vi "read from wavemeter_clock_2015.vi"(2 "error in (no error)":errorcluster, 3 "Single Measurement?":bool, 4 "Select Port":refnum<visa-resource-name>="COM4") -> (0 "error out":errorcluster, 1 "frequency":string="010849.313", 5 "Units":string=" cm-1")   [LabVIEW 2016]
uses:
  <vilib>/Instr/_visa.llb/VISA Configure Serial Port (Instr).vi
panel:
  in  "Case Constant\n(See Context Help) 2":bool=TRUE
  in  "Case Constant\n(See Context Help)":bool
  in  "termination char\n(0xA = '\\n' = LF)":u8=10 format="%.0x"
  in  "Tab Control":enum32{"Wavelength Monitor", "Nuts and Bolts"}(tab)
  out "Timestamp":string="17:39:12"
  out "Frequency":string="325253.97  GHz"
  out "Wavenumber":string="921.7173  nm"
  out "Wavelength":string="+010849.313  cm-1"
  out "Command String Sent":string
  in  "Send Command to Wavemeter":u16(ring) items=["Broadcast", "Deviation On", "Query", "Deviation off", "0", "1", "2", "3", "4", "5", "6", "7", "8", "9", "Clear", ".", "Enter", "Remote", "Save", "Reset", "Manual Deattenuate", "Manual Attenuate", "Auto Attenuate", "Humidity", "Pressure", "Temperature", "# Averaged", "Analog Res", "Display Res", "Setpoint", "Units", "Display", "Medium", "Resolution", "Averaging"]
  out "Array":dbl[](array[numeric])=[10849.313, 10849.313, 10849.313, 10849.313, 10849.313, 10849.313, 10849.313, 10849.313, 10849.313, 10849.313, 10849.313, 10849.313, 10849.313, 10849.313, 10849.313, 10849.313, 10849.314, 10849.313, 10849.313, 10849.313, 10849.313, 10849.313, 10849.313, 10849.313, 10849.313, 10849.313, 10849.313, 10849.313] format="%.4f"
  out "return count":u32=7
  out "Wavemeter Front Panel Values":T1={"Quantity"="010849.313 cm-1", "Uncertainty is:"="LOW", "Averaging ON?"=FALSE, "Resolution:"="FIXED"}
  out "Array of\nbuffer \noutputs":string[](array[string])=["+010849.313,2652,0200\r\n", "+010849.313,2652,0200\r\n", "+010849.313,2652,0200\r\n", "+010849.313,2652,0200\r\n", "+010849.313,2652,0200\r\n", "+010849.313,2652,0200\r\n", "+010849.313,2652,0200\r\n", "+010849.313,2652,0200\r\n", "+010849.313,2652,0200\r\n", "+010849.313,2652,0200\r\n", "+010849.313,2652,0200\r\n", "+010849.313,2652,0200\r\n", "+010849.313,2652,0200\r\n", "+010849.313,2652,0200\r\n", "+010849.313,2652,0200\r\n", "+010849.313,2652,0200\r\n", "+010849.314,2652,0200\r\n", "+010849.313,2652,0200\r\n", "+010849.313,2652,0200\r\n", "+010849.313,2652,0200\r\n", "+010849.313,2652,0200\r\n", "+010849.313,2652,0200\r\n", "+010849.313,2652,0200\r\n", "+010849.313,2652,0200\r\n", "+010849.313,2652,0200\r\n", "+010849.313,2652,0200\r\n", "+010849.313,2652,0200\r\n", "+010849.313,2652,0200\r\n"]
  out "Buffer output":string="+010849.313,2652,0200\r\n"
  # "COM4 For Radium"
  # "This stuff down here not useful for normal use.  Here \nfor trouble-shooting.  Feel free to ignore."
  # "Make sure RS232 cable is plugged into\nsecond COM port (COM2) on back of \nBarium.  If you want to use COM1, you\nneed to change it on the back panel of\nthis VI."
  # "Writing commands to wavemeter does \nnot currently work.  Still in the trouble-\nshooting process.  Read will work fine."
  # "This is quantity passed to calling VI."
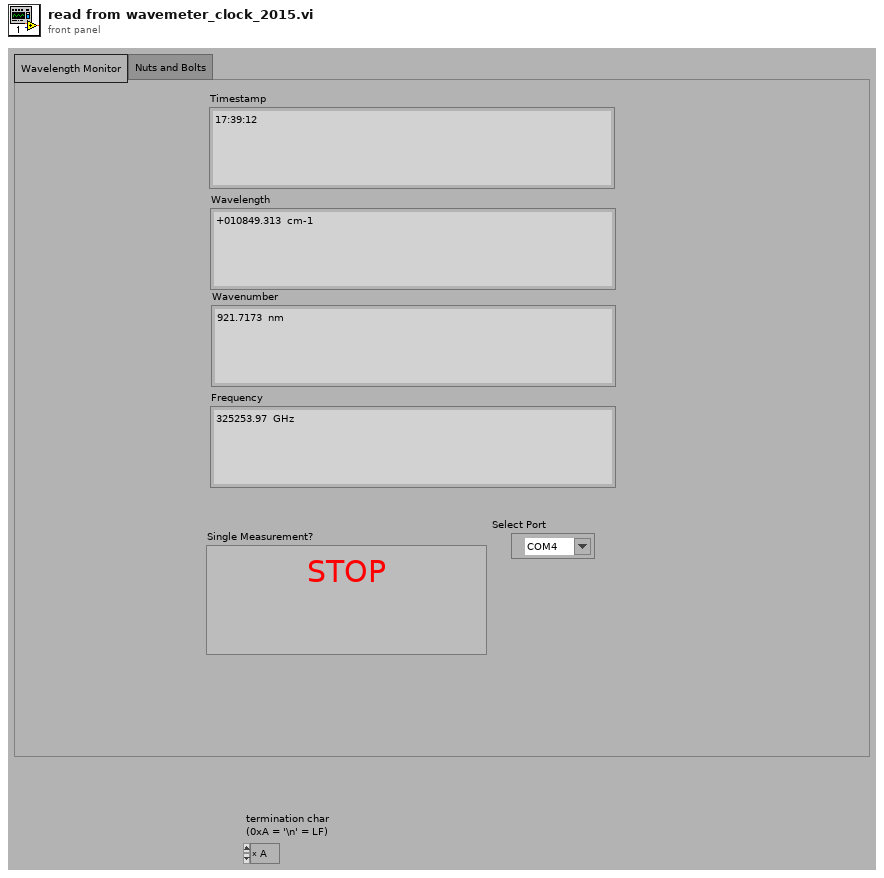
[diagram p1: front panel]
types:
  T1 = cluster{"Quantity":string, "Uncertainty is:":string, "Averaging ON?":bool, "Resolution:":string}
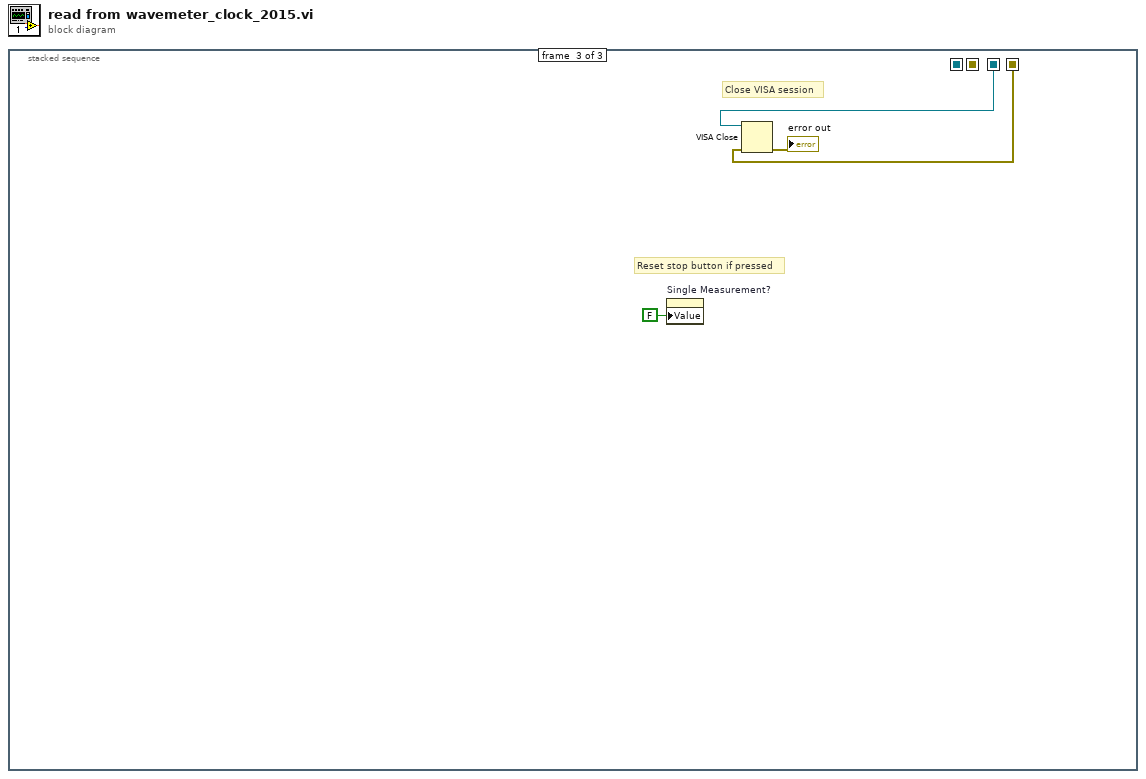
[diagram p0: block diagram]
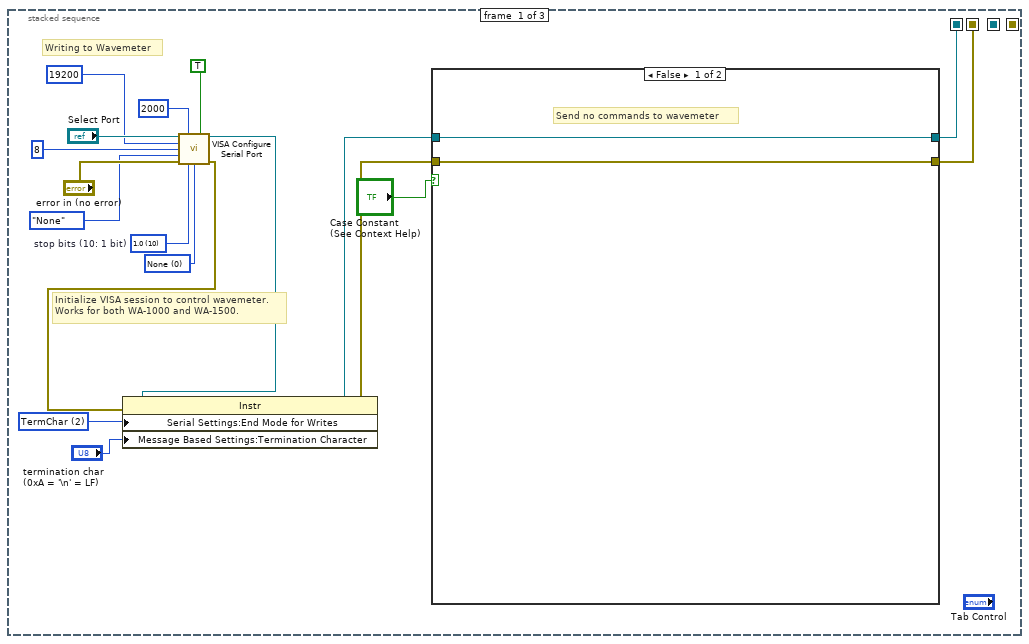
[diagram p2: hidden frame]
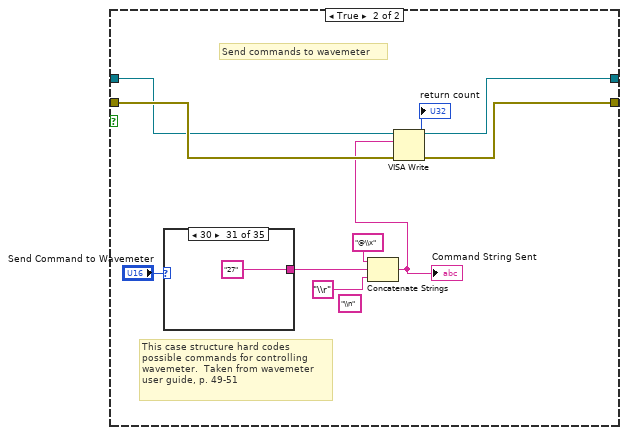
[diagram p3: hidden frame]
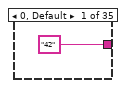
[diagram p4: hidden frame]
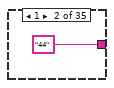
[diagram p5: hidden frame]
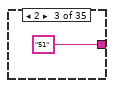
[diagram p6: hidden frame]
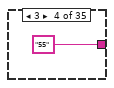
[diagram p7: hidden frame]
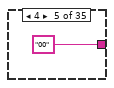
[diagram p8: hidden frame]
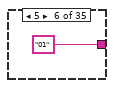
[diagram p9: hidden frame]
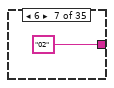
[diagram p10: hidden frame]
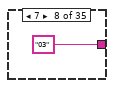
[diagram p11: hidden frame]
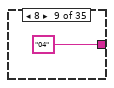
[diagram p12: hidden frame]
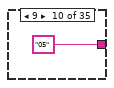
[diagram p13: hidden frame]
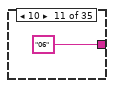
[diagram p14: hidden frame]
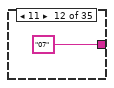
[diagram p15: hidden frame]
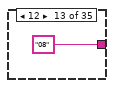
[diagram p16: hidden frame]
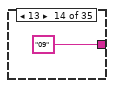
[diagram p17: hidden frame]
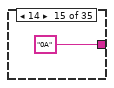
[diagram p18: hidden frame]
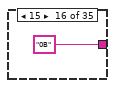
[diagram p19: hidden frame]
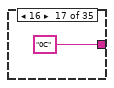
[diagram p20: hidden frame]
diagram:
  n1 = stacked-sequence {
    seq-local: [w17 _ _] -> [_ w70 _]
    seq-local: [w18 _ _] -> [_ w71 _]
    seq-local: [_ w68 _] -> [_ _ w221]
    seq-local: [_ w69 _] -> [_ _ w220]
    frame #0 {
      w2 = u16 2 items=["None", "LastBit", "TermChar", "Break"] ("Serial Settings:Serial End Mode for Writes")
      w8 = u16 0 items=["None"=0, "XON/XOFF"=1, "RTS/CTS"=2, "DTR/DSR"=4] ("flow control (0:none)")
      w9 = u16 10 items=["1.0"=10, "1.5"=15, "2.0"=20]  # stop bits (10: 1 bit)
      # "Initialize VISA session to control wavemeter.\nWorks for both WA-1000 and WA-1500."
      # "Writing to Wavemeter"
      n2 = call-poly "VISA Configure Serial Port"("VISA resource name"="Select Port", "timeout (10sec)"=u32 2000, "Enable Termination\nChar (T)"=TRUE ("Enable Termination\nChar (T)"), "baud rate (9600)"=u32 19200, "data bits (8)"=u16 8, "parity (0:none)"=enum16{"None", "Odd", "Even", "Mark", "Space"}."None", "error in (no error)"="error in (no error)", "stop bits (10: 1 bit)"=w9, "flow control (0:none)"=w8) -> ("VISA resource name out"=w6:refnum<visa-resource-name>, "error out"=w5:errorcluster)  [unwired: 5 in]
      n3 = property class="Instr"(reference=w6, error in=w5, "Serial Settings:End Mode for Writes"=w2, "Message Based Settings:Termination Character"="termination char\n(0xA = '\\n' = LF)") -> (reference out=w3:refnum<visa-resource-name>, error out=w4:errorcluster)
      n4 = case shown="False" "Case Constant\n(See Context Help)" {
        tunnel: w4 -> [w19 w30]
        tunnel: [w19 w25] -> w18
        tunnel: [w20 w27] -> w17
        tunnel: w3 -> [w20 w29]
        frame False {
          # "Send no commands to wavemeter"
        }
        frame True {
          (unwired) "\\n" ("string")
          # "This case structure hard codes\npossible commands for controlling\nwavemeter.  Taken from wavemeter\nuser guide, p. 49-51"
          # "Send commands to wavemeter"
          n5 = case shown="30" "Send Command to Wavemeter" {
            tunnel: ["42" "44" "51" "55" "00" "01" "02" "03" "04" "05" "06" "07" "08" "09" "0A" "0B" "0C" "0D" "0E" "0F" "10" "11" "13" "20" "21" "22" "23" "24" "25" "26" "27" "28" "29" "2A" "2B"] -> w21
            frame 0, Default {
            }
            frame 1 {
            }
            frame 2 {
            }
            frame 3 {
            }
            frame 4 {
            }
            frame 5 {
            }
            frame 6 {
            }
            frame 7 {
            }
            frame 8 {
            }
            frame 9 {
            }
            frame 10 {
            }
            frame 11 {
            }
            frame 12 {
            }
            frame 13 {
            }
            frame 14 {
            }
            frame 15 {
            }
            frame 16 {
            }
            frame 17 {
            }
            frame 18 {
            }
            frame 19 {
            }
            frame 20 {
            }
            frame 21 {
            }
            frame 22 {
            }
            frame 23 {
            }
            frame 24 {
            }
            frame 25 {
            }
            frame 26 {
            }
            frame 27 {
            }
            frame 28 {
            }
            frame 29 {
            }
            frame 30 {
            }
            frame 31 {
            }
            frame 32 {
            }
            frame 33 {
            }
            frame 34 {
            }
          }
          n6 = Concatenate Strings("@\\x", w21, "\\r" ("string")) -> (w22:string)
          "Command String Sent" <- w22
          n7 = VISA Write(VISA resource name=w29, write buffer=w22, error in (no error)=w30) -> (VISA resource name out=w27:refnum<visa-resource-name>, return count=→"return count":u32, error out=w25:errorcluster)
        }
      }
    }
    frame #1 {
      w66 = ext 299792224.68100000001  # speed of light for freq. conversion
      # "Wavemeter should\nbe in broadcast mode\nin order for this section\nto work correctly.\n\nIn broadcast mode,\nwavemeter announces\nfront panel reading\nperiodically and this \ncode parses that string\nand displays the\nwavelength."
      n8 = case shown="True" "Case Constant\n(See Context Help) 2" {
        tunnel: w71 -> [w73 w82]
        tunnel: w70 -> [w72 w81]
        tunnel: [w73 w80] -> w69
        tunnel: [w72 w79] -> w68
        tunnel: w66 -> [_ w74]
        frame False {
          # "Don't read from wavemeter."
        }
        frame True {
          # "Read from\nwavemeter"
          n9 = while {
            tunnel: w81 -> [w116]
            tunnel: w82 -> [w115]
            tunnel: [w113] -> w80
            tunnel: [w112] -> w79
            shift-right: [w111] -> w77
            shift-left: string[] [] -> [w110]
            shift-right: [w104] -> w75
            shift-left: dbl[] [] -> [w103]
            tunnel: w74 -> [w91]
            stop <- "Single Measurement?" stop-if-true
            w100 = ","  # search string/char (-)
            # "Delay between measurements.\nAdjust to have fewer data points saved."
            n10 = VISA Read(VISA resource name=w116, byte count=u32 23 ("byte count (0)"), error in (no error)=w115) -> (VISA resource name out=w112:refnum<visa-resource-name>, read buffer=w101:string, error out=w113:errorcluster)  [unwired: 1 out]
            "Buffer output" <- w101
            n11 = Build Array (concatenate)(w110, w101) -> (w111:string[])
            n12 = Spreadsheet String To Array(delimiter (Tab)="\\n", format string="%s", spreadsheet string=w101, array type (2D Dbl)=string[] []) -> (array=w105:string[])
            n13 = Search/Split String(string=w101, search string/char (-)=w100, offset (0)=1) -> (substring before match=w90:string, match + rest of string=w98:string)  [unwired: 1 out]
            n14 = for {
              tunnel: w105 -> [w173] mode=indexing
              tunnel: [w172] -> w102 mode=indexing
              i -> [w174]
              n15 = case shown="0, Default" w174 {
                tunnel: w173 -> [w180 w210 _]
                tunnel: [w177 _ _] -> w172
                frame 0, Default {
                  n16 = String Subset "Uncertainty"(string=w180, length (rest)=1 ("length (rest)")) -> (substring=w200:string)  [unwired: 1 in]
                  n17 = String Subset "Averaging Status"(string=w180, offset (0)=12, length (rest)=1 ("length (rest)")) -> (substring=w196:string)
                  n18 = String Subset "Units of Wavelength"(string=w180, offset (0)=15, length (rest)=1 ("length (rest)")) -> (substring=w192:string)
                  n19 = String Subset "Fixed or Auto Resolution"(string=w180, offset (0)=13, length (rest)=1 ("length (rest)")) -> (substring=w182:string)
                  n20 = Equal?(x="~", y=w200) -> (x = y?=w202:bool)
                  n21 = case shown="False" w202 {
                    tunnel: ["LOW" "HIGH"] -> w187
                    frame False {
                    }
                    frame True {
                    }
                  }
                  n22 = Decimal String To Number(string=w192) -> (number=w191:i32)  [unwired: 2 in, 1 out]
                  n23 = Equal?(x="1", y=w196) -> (x = y?=w186:bool)
                  n24 = Equal?(x="A", y=w182) -> (x = y?=w179:bool)
                  n25 = case shown="4" w191 {
                    tunnel: [_ " cm-1" " GHz" " nm"] -> w188
                    frame 0, Default {
                    }
                    frame 2 {
                    }
                    frame 4 {
                    }
                    frame 9 {
                    }
                  }
                  "Units" <- w188
                  n26 = case shown="False" w179 {
                    tunnel: ["FIXED" "AUTO"] -> w178
                    frame False {
                    }
                    frame True {
                    }
                  }
                  n27 = String Subset "Wavelength"(string=w180, offset (0)=1, length (rest)=10 ("length (rest)")) -> (substring=w175:string)
                  "frequency" <- w175
                  n28 = Concatenate Strings(w175, w188) -> (w176:string)
                  n29 = Bundle(w176, w187, w186, w178) -> (→"Wavemeter Front Panel Values":cluster{string, string, bool, string})  [unwired: 1 in]
                  n30 = Scan From String(input string=w175) -> (output 1=w177:dbl)  [unwired: 4 in, 3 out]
                }
                frame 1 {
                  n31 = String Subset "Averaging On/Off"(string=w210, offset (0)=0, length (rest)=1 ("length (rest)")) -> ()  [unwired: 1 out]
                  n32 = String Subset "Quantity"(string=w210, offset (0)=2, length (rest)=1 ("length (rest)")) -> ()  [unwired: 1 out]
                  n33 = String Subset "Quantity"(string=w210, offset (0)=3, length (rest)=1 ("length (rest)")) -> ()  [unwired: 1 out]
                  n34 = String Subset "Quantity"(string=w210, offset (0)=1, length (rest)=1 ("length (rest)")) -> ()  [unwired: 1 out]
                }
                frame 2 {
                }
              }
            }
            n35 = String Subset(string=w98, offset (0)=1, length (rest)=4 ("length (rest)")) -> (substring=w88:string)
            n36 = Fract/Exp String To Number(string=w88) -> (number=w87:dbl)  [unwired: 3 in, 1 out]
            n37 = Fract/Exp String To Number(string=w90) -> (number=w89:dbl)  [unwired: 3 in, 1 out]
            n38 = case shown="0, Default" w87 {
              tunnel: [w117 w135 w145 w154] -> w95
              tunnel: [w117 w128 w152 w155] -> w94
              tunnel: [w117 w122 w143 w156] -> w93
              tunnel: w90 -> [_ w133 w151 w170]
              tunnel: w89 -> [_ w124 w150 w169]
              tunnel: 1e-07 ("x") -> [_ w126 w148 w161]
              tunnel: w91 -> [_ w125 w138 w168]
              frame 0, Default {
                w117 = "No measurement"
              }
              frame 2649 {
                w120 = "  "
                n39 = Multiply(x=w126, y=w124) -> (x*y=w132:dbl)
                n40 = Concatenate Strings(w133, w120, "nm" ("string")) -> (w135:string)
                n41 = Reciprocal(x=w132) -> (1/x=w131:dbl)
                n42 = Number To Fractional String(number=w131, precision (6)=i16 3) -> (F-format string=w130:string)  [unwired: 2 in]
                n43 = Divide(x=w125, y=w124) -> (x/y=w123:ext)
                n44 = Concatenate Strings(w130, w120, "cm-1" ("string")) -> (w128:string)
                n45 = Number To Fractional String(number=w123, precision (6)=i16 2) -> (F-format string=w121:string)  [unwired: 2 in]
                n46 = Concatenate Strings(w121, w120, "GHz" ("string")) -> (w122:string)
              }
              frame 2652 {
                w141 = "  " ("string")
                n47 = Reciprocal(x=w150) -> (1/x=w149:dbl)
                n48 = Divide(x=w149, y=w148) -> (x/y=w139:dbl)
                n49 = Concatenate Strings(w151, w141, "cm-1" ("string")) -> (w152:string)
                n50 = Number To Fractional String(number=w139, precision (6)=i16 4) -> (F-format string=w147:string)  [unwired: 2 in]
                n51 = Divide(x=w138, y=w139) -> (x/y=w140:ext)
                n52 = Concatenate Strings(w147, w141, "nm" ("string")) -> (w145:string)
                n53 = Number To Fractional String(number=w140, precision (6)=i16 2) -> (F-format string=w142:string)  [unwired: 2 in]
                n54 = Concatenate Strings(w142, w141, "GHz" ("string")) -> (w143:string)
              }
              frame 2664 {
                w157 = "  " ("string")
                n55 = Concatenate Strings(w170, w157, "GHz" ("string")) -> (w156:string)
                n56 = Divide(x=w169, y=w168) -> (x/y=w160:ext)
                n57 = Reciprocal(x=w160) -> (1/x=w164:ext)
                n58 = Number To Fractional String(number=w164, precision (6)=i16 4) -> (F-format string=w165:string)  [unwired: 2 in]
                n59 = Divide(x=w160, y=w161) -> (x/y=w162:ext)
                n60 = Concatenate Strings(w165, w157, "nm" ("string")) -> (w155:string)
                n61 = Number To Fractional String(number=w162, precision (6)=i16 3) -> (F-format string=w166:string)  [unwired: 2 in]
                n62 = Concatenate Strings(w166, w157, "cm-1" ("string")) -> (w154:string)
              }
            }
            "Wavelength" <- w94
            "Wavenumber" <- w95
            "Frequency" <- w93
            n63 = Get Date/Time In Seconds() -> (seconds since 1Jan1904=w84:timestamp)
            n64 = Build Array (concatenate)(w103, w102) -> (w104:dbl[])
            n65 = Format Date/Time String(time format string (%c)="%H:%M:%S", seconds (now)=w84) -> (date/time string=→"Timestamp":string)  [unwired: 1 in]
            n66 = Wait (ms)(milliseconds to wait=u32 0) -> ()  [unwired: 1 out]
          }
          "Array of\nbuffer \noutputs" <- w77
          "Array" <- w75
        }
      }
    }
    frame #2 {
      # "Reset stop button if pressed"
      # "Close VISA session"
      n67 = property on="Single Measurement?" class="Bool (strict)"("Value"=FALSE ("Single Measurement?")) -> ()  [unwired: 2 in, 2 out]
      n68 = VISA Close(VISA resource name=w221, error in (no error)=w220) -> (error out=→"error out":errorcluster)
    }
  }
